vi "Graph Cursors.vi"() -> ()   [LabVIEW 2023]
doc: "This example demonstrates how to programmatically change the values of cursors. Three types of cursors are demonstrated, Single-Plot, Multi-Plot and Free Cursors. They are shown on a graph with two different random plots."
panel:
  out "Mixed Signal Graph":dbl[][](graph)
  # "Overview: Demonstrates the use of Graph Cursors to navigate the data within a graph.\nInstructions:\nRun the VI. Cursors will appear within the graph with the following characteristics:\n\nCursor 0 - Free cursor that can be moved anywhere within the plot area.\nCursor 1 - Multi-plot cursor that can be positioned along any of the plots within Group 0 of the graph.\nCursor 2 - Single-plot cursor that can be positioned along Plot 0 only."
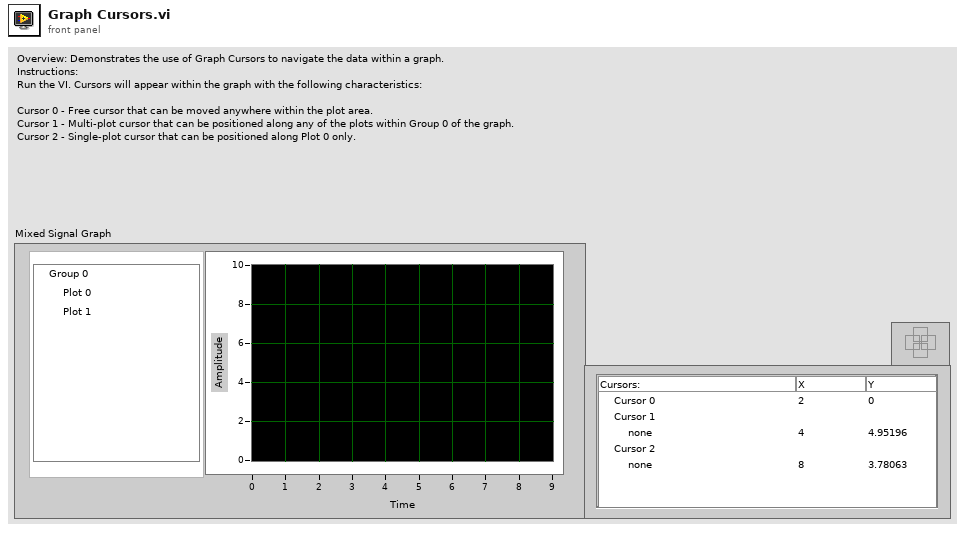
[diagram p1: front panel]
types:
  T1 = typedef "LVCursorListTypeDef.ctl" = cluster{"Name":string, "Color":u32, "Style":u8, "Point Style":u8, "Name Visible":bool, "Allow Drag":bool, "Cursor Mode":u32, "Plot":i32, "Index":i32, "Position":cluster{"X":dbl, "Y":dbl}, "X Scale":u32, "Y Scale":u32, "Watch Plots":i32[], "Watch All Plots":bool, "Plot Area":i32, "Label Offset":cluster{"X":dbl, "Y":dbl}}[]
  T2 = cluster{"Name":string, "Color":u32, "Style":u8, "Point Style":u8, "Name Visible":bool, "Allow Drag":bool, "Cursor Mode":u32, "Plot":i32, "Index":i32, "Position":cluster{"X":dbl, "Y":dbl}, "X Scale":u32, "Y Scale":u32, "Watch Plots":i32[], "Watch All Plots":bool, "Plot Area":i32, "Label Offset":cluster{"X":dbl, "Y":dbl}}
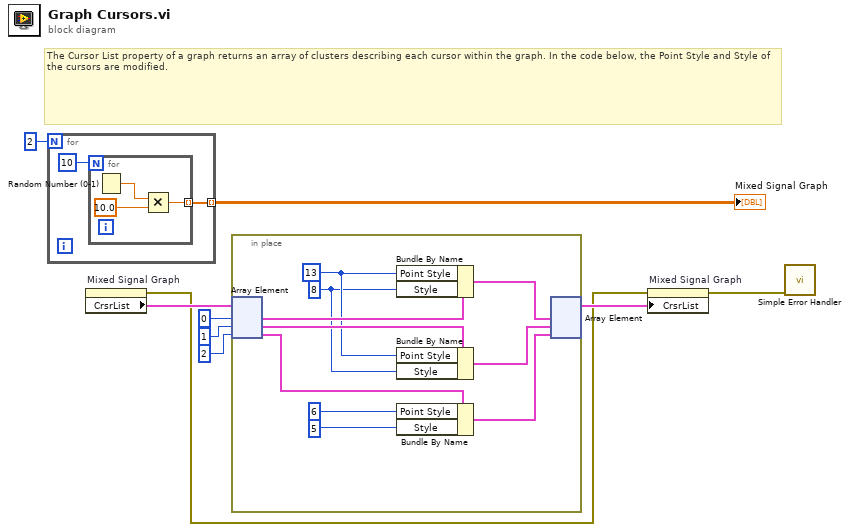
[diagram p0: block diagram]
diagram:
  # "The Cursor List property of a graph returns an array of clusters describing each cursor within the graph. In the code below, the Point Style and Style of the cursors are modified."
  n1 = for {
    N: 2 -> [_]
    tunnel: [w10] -> w3 mode=indexing
    n2 = for {
      N: 10 -> [_]
      tunnel: [w12] -> w10 mode=indexing
      n3 = Random Number (0-1)() -> (number: 0 to 1=w13:dbl)
      n4 = Multiply(x=w13, y=10.0) -> (x*y=w12:dbl)
    }
  }
  "Mixed Signal Graph" <- w3
  n5 = property on="Mixed Signal Graph" class="MixedSignalGraph (strict)"() -> (error out=w1:errorcluster, "CrsrList"=w4:T1)  [unwired: 2 in, 1 out]
  n6 = in-place {
    w20 = u8 8
    w21 = u8 13
    n7 = in-place-array #1(w4, 0, 1, 2) -> (w24:T2, w22:T2, w18:T2)
    n8 = Bundle By Name(cluster=w24, "Point Style"=w21, "Style"=w20) -> (w23:T2)
    n9 = Bundle By Name(cluster=w22, "Point Style"=w21, "Style"=w20) -> (w19:T2)
    n10 = Bundle By Name(cluster=w18, "Point Style"=u8 6, "Style"=u8 5) -> (w17:T2)
    n11 = in-place-array #1(w23, w19, w17) -> (w8:T1)  [unwired: 3 out]
  }
  n12 = property on="Mixed Signal Graph" class="MixedSignalGraph (strict)"(error in=w1, "CrsrList"=w8) -> (error out=w2:errorcluster)  [unwired: 1 in, 1 out]
  n13 = call <vilib>:"Simple Error Handler.vi"("error in (no error)"=w2) -> ()  [unwired: 4 in, 5 out]
